vi "Message Globals.vi"() -> ()   [LabVIEW 2021]
panel:
  in  "Invalid Callback Path":string="Path contains invalid characters. Acceptable characters: letters, numbers, spaces and _+-!@#$%^()[]{};'~`,. "
  in  "Broken Callback Error":string="The callback VI is broken."
  in  "Broken Callback Error Details":string="The callback VI is broken. Make sure the callback VI is executable in order to run an Interrupt Express VI."
  in  "Callback Error":string="The callback VI path is not specified."
  in  "File not found":string="The callback VI is not found. Ensure that the path you specify for the callback VI is correct."
  in  "Unconfigurate Callback":string="You did not specify a path to the callback VI in the Expess VI configuration dialog box."
  in  "Callback not Found":string="The callback VI is not found. The expected callback VI path is %s."
  in  "Create Callback Prompt":string="Specify a name for the callback VI"
  in  "No VI Ext":string="The specified file path is not a VI. Specify a callback VI path."
  in  "Select Callback Prompt":string="Select an existing callback VI"
  in  "No Permission":string="The callback VI was not created because you do not have permission to save the callback VI in this directory.\n\nOpen the Express VI and specify a different callback VI path."
  in  "Empty Path":string="Specify a callback VI path."
  in  "Name Used":string="The callback VI name is duplicated with a VI in memory or in the project. Specify a different callback VI."
  in  "Connector Not Match":string="The connector pane of this VI does not meet callback VI requirements."
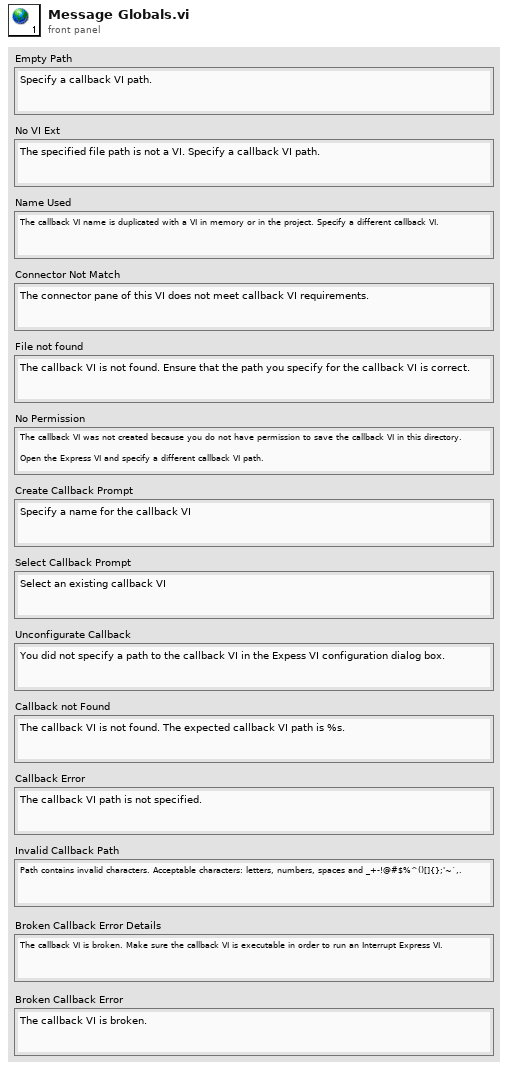
[diagram p1: front panel]
diagram:
